vi "Init.vi"(3 "Container State":T3, 4 "Previous State":variant, 5 "Previous Version":T2) -> (2 "Current State":T1={"Pin Disabled?"=[enum."Enabled", enum."Enabled", enum."Enabled", enum."Enabled", enum."Enabled", enum."Enabled", enum."Enabled", enum."Enabled", enum."Enabled", enum."Enabled", enum."Enabled", enum."Enabled", enum."Enabled", enum."Enabled", enum."Enabled", enum."Enabled", enum."Enabled", enum."Enabled", enum."Enabled", enum."Enabled"], "Pin Name"=["", "", "", "", "", "", "", "", "", "", "", "", "", "", "", "", "", "", "", ""], "Pin ID"=["0", "1", "2", "3", "4", "5", "6", "7", "8", "9", "10", "11", "12", "13", "14", "15", "16", "17", "18", "19"], "Connector Name"="DIO", "Row Name 1"="S", "Row Name 2"="5V"})   [LabVIEW 2021, in "roboRIO 10 Bank.xctl"]
uses:
  <vilib>/myRIO/Common/Instrument Driver Framework/Utilities/xctls/roboRIO 10 Bank/roboRIO 10 Bank.xctl
  <vilib>/myRIO/Common/Instrument Driver Framework/Utilities/xctls/roboRIO 10 Bank/State.ctl
  <vilib>/_xctls/Container State.ctl
  <vilib>/_xctls/Version.ctl
  <vilib>/_xctls/XControlSupport.lvlib
panel:
  in  "Default Indicator State":T1={"Pin Disabled?"=[enum."Enabled", enum."Enabled", enum."Enabled", enum."Enabled", enum."Enabled", enum."Enabled", enum."Enabled", enum."Enabled", enum."Enabled", enum."Enabled", enum."Enabled", enum."Enabled", enum."Enabled", enum."Enabled", enum."Enabled", enum."Enabled", enum."Enabled", enum."Enabled", enum."Enabled", enum."Enabled"], "Pin Name"=["", "", "", "", "", "", "", "", "", "", "", "", "", "", "", "", "", "", "", ""], "Pin ID"=["0", "1", "2", "3", "4", "5", "6", "7", "8", "9", "10", "11", "12", "13", "14", "15", "16", "17", "18", "19"], "Connector Name"="DIO", "Row Name 1"="S", "Row Name 2"="5V"}
  in  "Default Control State":T1={"Pin Disabled?"=[enum."Enabled", enum."Enabled", enum."Enabled", enum."Enabled", enum."Enabled", enum."Enabled", enum."Enabled", enum."Enabled", enum."Enabled", enum."Enabled", enum."Enabled", enum."Enabled", enum."Enabled", enum."Enabled", enum."Enabled", enum."Enabled", enum."Enabled", enum."Enabled", enum."Enabled", enum."Enabled"], "Pin Name"=["", "", "", "", "", "", "", "", "", "", "", "", "", "", "", "", "", "", "", ""], "Pin ID"=["0", "1", "2", "3", "4", "5", "6", "7", "8", "9", "10", "11", "12", "13", "14", "15", "16", "17", "18", "19"], "Connector Name"="DIO", "Row Name 1"="S", "Row Name 2"="5V"}
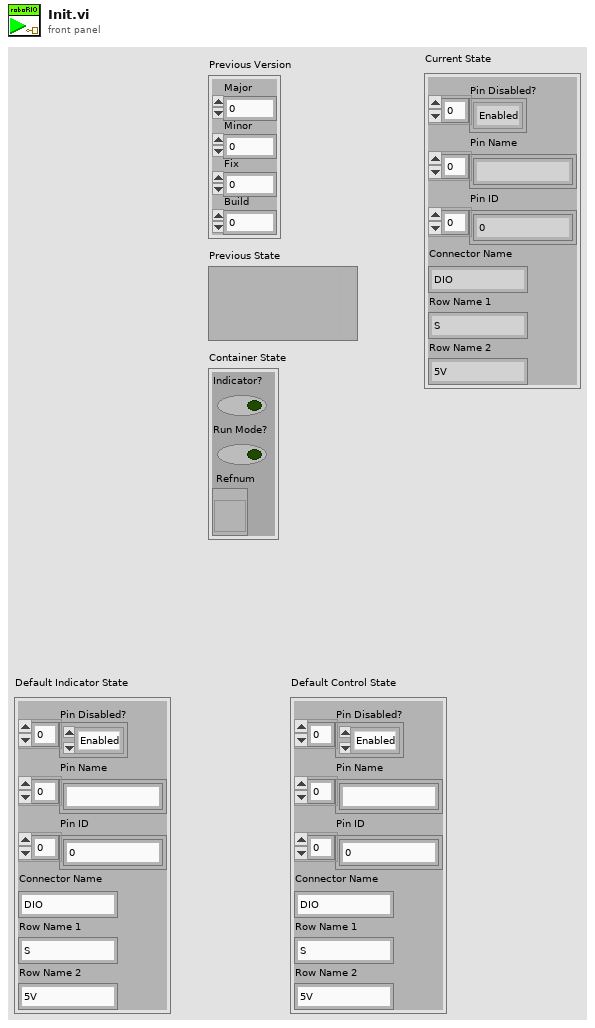
[diagram p1: front panel]
types:
  T1 = typedef "roboRIO 10 Bank.xctl/State.ctl" = cluster{"Pin Disabled?":enum8{"Enabled", "Disabled", "Disabled and Grayed Out"}[], "Pin Name":string[], "Pin ID":string[], "Connector Name":string, "Row Name 1":string, "Row Name 2":string}
  T2 = typedef "XControlSupport.lvlib/Version.ctl" = cluster{"Major":u16, "Minor":u16, "Fix":u16, "Build":u16}
  T3 = typedef "XControlSupport.lvlib/Container State.ctl" = cluster{"Indicator?":bool, "Run Mode?":bool, " Refnum":refnum<vi>}
  T4 = enum8{"Enabled", "Disabled", "Disabled and Grayed Out"}[]
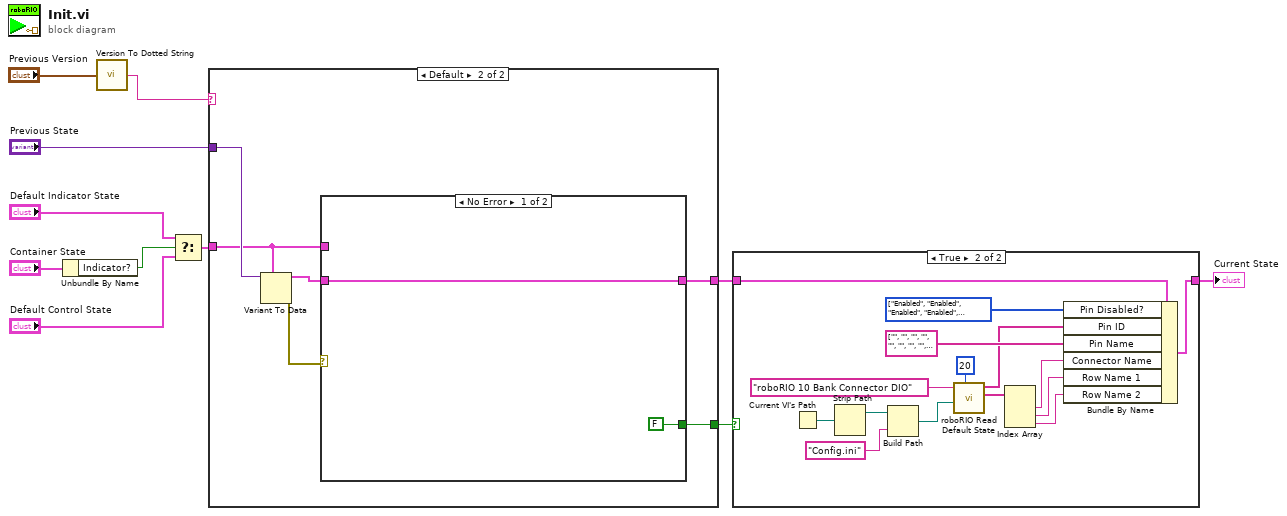
[diagram p0: block diagram]
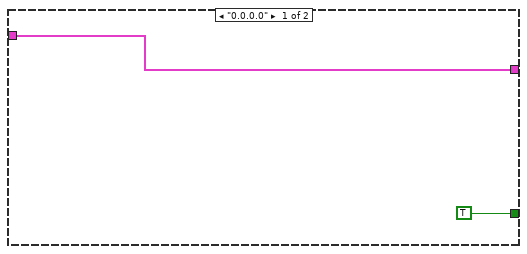
[diagram p3: hidden frame]
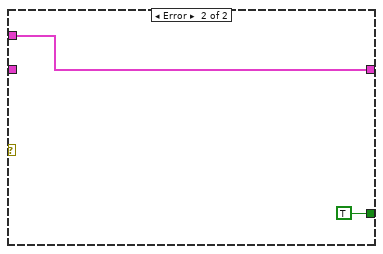
[diagram p4: hidden frame]
diagram:
  n1 = Unbundle By Name("Container State") -> ("Indicator?"=w7:bool)
  n2 = call <vilib>:"Version To Dotted String.vi"("Version"="Previous Version") -> ("String Version"=w4:string)
  n3 = Select(t="Default Indicator State", s=w7, f="Default Control State") -> (s? t:f=w6:T1)
  n4 = case shown="Default" w4 {
    tunnel: "Previous State" -> [_ w19]
    tunnel: [w13 w15] -> w2
    tunnel: w6 -> [w13 w16]
    tunnel: [TRUE w14] -> w3
    frame "0.0.0.0" {
    }
    frame Default {
      n5 = Variant To Data(type=w16, Variant=w19) -> (data=w17:T1, error out=w18:errorcluster)  [unwired: 1 in]
      n6 = case shown="No Error" w18 {
        tunnel: w17 -> [w21 _]
        tunnel: [w21 w22] -> w15
        tunnel: w16 -> [_ w22]
        tunnel: [FALSE TRUE] -> w14
        frame No Error {
        }
        frame Error {
        }
      }
    }
  }
  n7 = case shown="True" w3 {
    tunnel: w2 -> [w24 w26]
    tunnel: [w24 w25] -> w1
    frame False {
    }
    frame True {
      w39 = T4 [enum."Enabled", enum."Enabled", enum."Enabled", enum."Enabled", enum."Enabled", enum."Enabled", enum."Enabled", enum."Enabled", enum."Enabled", enum."Enabled", enum."Enabled", enum."Enabled", enum."Enabled", enum."Enabled", enum."Enabled", enum."Enabled", enum."Enabled", enum."Enabled", enum."Enabled", enum."Enabled"] items=["Enabled", "Disabled", "Disabled and Grayed Out"] ("subarray")
      n8 = Current VI's Path() -> (path=w29:path)
      n9 = Strip Path(path=w29) -> (stripped path=w28:path)  [unwired: 1 out]
      n10 = Build Path(base path=w28, name or relative path="Config.ini") -> (appended path=w32:path)
      n11 = call <vilib>:"roboRIO Read Default State.vi"("Size"=20, "Path"=w32, "Connector"="roboRIO 10 Bank Connector DIO") -> ("Default Connector Info"=w34:string[], "Default Pins IDs"=w33:string[])  [unwired: 6 in, 1 out]
      n12 = Index Array(array=w34) -> (element #1=w35:string, element #2=w36:string, element #3=w37:string)  [unwired: 3 in]
      n13 = Bundle By Name(cluster=w26, "Pin Disabled?"=w39, "Pin ID"=w33, "Pin Name"=string[] ["", "", "", "", "", "", "", "", "", "", "", "", "", "", "", "", "", "", "", ""] ("Pin Alias"), "Connector Name"=w35, "Row Name 1"=w36, "Row Name 2"=w37) -> (w25:T1)
    }
  }
  "Current State" <- w1
